vi "TEST Handle FGV User Event Reference Manager.vi"() -> ()   [LabVIEW 2011]
doc: "This is the second solution of a two VI test process for the FGV User Event Reference Manager. This VI handles the User Events that are fired.\n\nAAL 9/09"
uses:
  Type Defs/TYPE FGV User Event Method.ctl
panel:
  in  "Cancel":bool
  in  "OK":bool
  out "String":string
  out "Data":timestamp
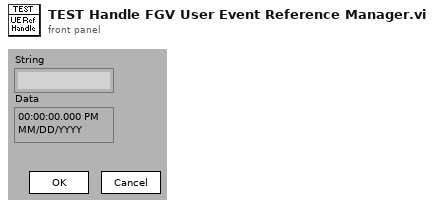
[diagram p1: front panel]
types:
  T1 = typedef "TYPE FGV User Event Method.ctl" = enum16{"Add User Event Ref", "Get User Event Ref", "Delete User Event Ref", "Get All User Event Refs", "Delete All User Event Refs"}
  T2 = typedef "TYPE FGV User Event Ref.ctl" = refnum<user-event>
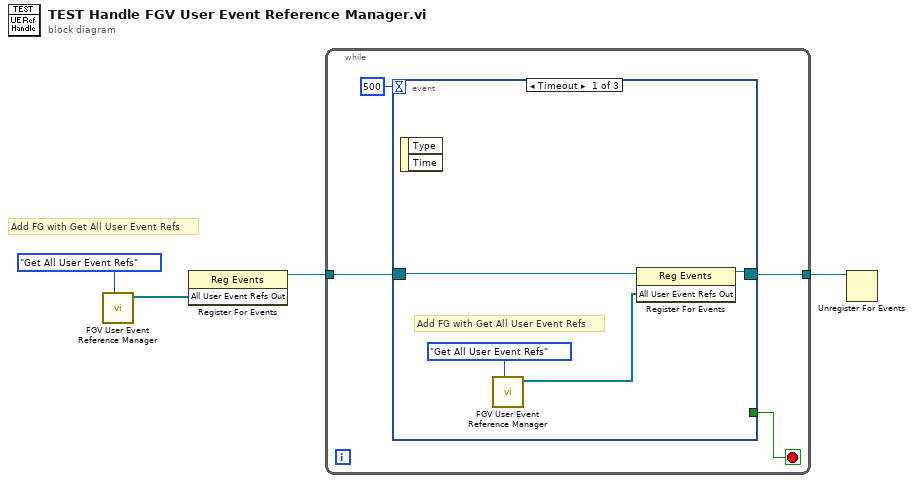
[diagram p0: block diagram]
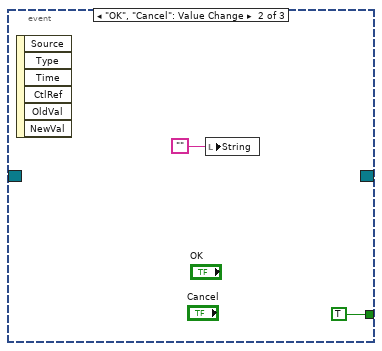
[diagram p2: hidden frame]
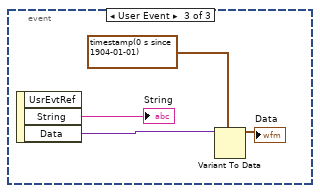
[diagram p3: hidden frame]
diagram:
  # "Add FG with Get All User Event Refs"
  n1 = call "FGV User Event Reference Manager.vi"("Method (Get User Event Ref)"=TYPE_FGV_User_Event_Method."Get All User Event Refs") -> ("All User Event Refs Out"=w1:T2[])  [unwired: 2 in, 8 out]
  n2 = register-events(w1) -> (reference out=w3:refnum<event-registration>)  [unwired: 2 in, 1 out]
  n3 = while {
    tunnel: w3 -> [w5]
    tunnel: [w7] -> w2
    stop <- w6 stop-if-true
    n4 = event shown="[0] Timeout" {
      selector: w5 -> [w11 _ _]
      dyn-events: [w10 _ _] -> w7
      timeout: 500 -> [_ _ _]
      tunnel: [_ TRUE ("stop") _] -> w6
      event Timeout {
        # "Add FG with Get All User Event Refs"
        n5 = event-data() -> ()  [unwired: 3 out]
        n6 = call "FGV User Event Reference Manager.vi"("Method (Get User Event Ref)"=TYPE_FGV_User_Event_Method."Get All User Event Refs") -> ("All User Event Refs Out"=w9:T2[])  [unwired: 2 in, 8 out]
        n7 = register-events(reference=w11, w9) -> (reference out=w10:refnum<event-registration>)  [unwired: 1 in, 1 out]
      }
      event "OK", "Cancel": Value Change {
        n8 = event-data() -> ()  [unwired: 7 out]
        n9 = local write "String"("") -> ()
      }
      event User Event {
        n10 = event-data() -> ("String"=→"String":string, "Data"=w16:variant)  [unwired: 2 out]
        n11 = Variant To Data(type=timestamp(0 s since 1904-01-01), Variant=w16) -> (data=→"Data":timestamp)  [unwired: 1 in, 1 out]
      }
    }
  }
  n12 = Unregister For Events(event registration refnum=w2) -> ()  [unwired: 1 in, 1 out]
